vi "校准任务流程.vi"(9 "校准任务":T1[](array[typedef]), 10 "精度":dbl=4.0, 11 "模型":enum32{"线性", "多项式", "折线"}(ring)) -> ()   [LabVIEW 2016, in "斯坦道CODMn.lvlib"]
uses:
  <userlib>/_OpenG.lib/array/array.llb/Remove Duplicates from 1D Array (U16)__ogtk.vi
panel:
  out "元素":T1
  out "执行列表":T2(ring)
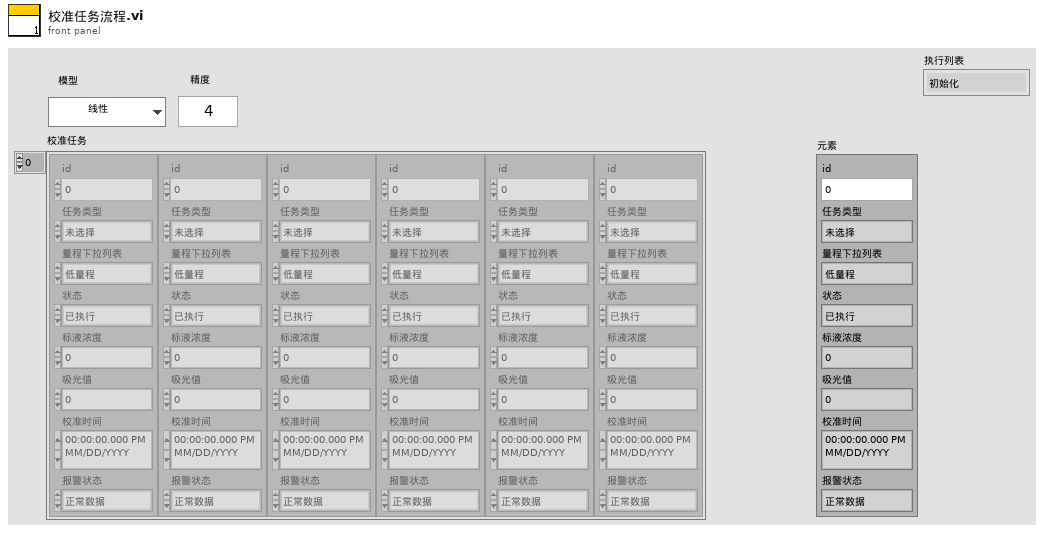
[diagram p1: front panel]
types:
  T1 = typedef "斯坦道CODMn.lvlib/校准任务.ctl" = cluster{"id":u16, "任务类型":enum16{"未选择", "空白校准", "标样校准", "标样核查", "零点核查", "跨度核查"}, "量程下拉列表":enum16{"低量程", "高量程"}, "状态":enum16{"已执行", "待执行", "执行中", "停止"}, "标液浓度":dbl, "吸光值":dbl, "校准时间":timestamp, "报警状态":enum16{"正常数据", "报警数据"}}
  T2 = enum16{"初始化", "解析数据", "判断任务类型", "执行测试任务", "等待测试任务完成", "获取测试数据", "任务结束判定", "计算公式", "结束"}
  T3 = cluster{"时间标识":timestamp, "设备":string, "日志信息":string, "流程参数":string}
  T4 = cluster{"测量模式":enum16{"水样测量", "标样核查", "零点核查", "跨度核查", "空白测试", "加标回收", "平行样", "校零", "校标"}}
  T5 = enum16{"水样测量", "标样核查", "零点核查", "跨度核查", "空白测试", "加标回收", "平行样", "校零", "校标"}
  T6 = cluster{"标液浓度1":dbl, "测量吸光度1":dbl, "样品1启用":bool, "标液浓度2":dbl, "测量吸光度2":dbl, "样品2启用":bool, "标液浓度3":dbl, "测量吸光度3":dbl, "样品3启用":bool, "标液浓度4":dbl, "测量吸光度4":dbl, "样品4启用":bool, "标液浓度5":dbl, "测量吸光度5":dbl, "样品5启用":bool, "模型":enum32{"线性", "多项式", "折线"}, "精度":dbl, "XY图":cluster{"X Values":dbl[], "Y Values":dbl[]}[], "拟合公式":string, "r^2":dbl, "标样一校准时间":timestamp, "标样二校准时间":timestamp, "标样三校准时间":timestamp, "标样四校准时间":timestamp, "标样五校准时间":timestamp, "二次方程":cluster{"c":dbl, "B":dbl, "x^2":dbl}, "标定时间":timestamp, "拟合公式 2":string, "r^2 2":dbl}
  T7 = enum16{"", "水样测量", "标样核查", "零点核查", "跨度核查", "空白测试", "平行样测试", "加标回收", "空白校准", "标样校准"}
  T8 = typedef "报警信息字段定义.ctl" = cluster{"时间":timestamp, "参数":string, "报警信息":string, "备注":string, "code":u64, "platform_alarm_code":string}
  T9 = cluster{"因子编码":u32, "单位":u16, "标样参考值":sgl, "水样数据时间":timestamp, "水样实测值":sgl, "水样数据标识":string, "标样数据时间":timestamp, "标样实测值":sgl, "标样数据标识":string, "空白数据时间":timestamp, "空白实测值":sgl, "空白数据标识":string, "零点核查数据时间":timestamp, "零点核查实测值":sgl, "零点核查数据标识":string, "跨度核查数据时间":timestamp, "跨度核查实测值":sgl, "跨度核查数据标识":string, "加标回收数据时间":timestamp, "加标回收实测值":sgl, "加标回收数据标识":string, "平行样数据时间":timestamp, "平行样实测值":sgl, "平行样数据标识":string}
  T10 = cluster{"时间":timestamp, "测量模式":string, "数据类型":string, "检测值":sgl, "单位":string, "数据标识":string, "因子编码":string, "标样参考值":sgl, "ORP-A":sgl, "ORP-B":sgl, "ORP-K":sgl, "COD滴定值":sgl, "高锰酸钾滴定数":sgl, "温度":sgl, "量程":sgl, "LastTime":timestamp, "序列号:":string, "跨度值":sgl, "高锰酸钾原始滴定数":sgl, "F0":sgl, "F1":sgl, "F2":sgl, "F3":sgl, "F4":sgl, "F5":sgl, "启动温度":sgl}
  T11 = enum16{"未选择", "空白校准", "标样校准", "标样核查", "零点核查", "跨度核查"}
  T12 = cluster{"标液浓度1":dbl, "测量吸光度1":dbl, "样品1启用":bool, "标液浓度2":dbl, "测量吸光度2":dbl, "样品2启用":bool, "标液浓度3":dbl, "测量吸光度3":dbl, "样品3启用":bool, "标液浓度4":dbl, "测量吸光度4":dbl, "样品4启用":bool, "标液浓度5":dbl, "测量吸光度5":dbl, "样品5启用":bool, "模型":enum32{"线性", "多项式", "折线"}, "精度":dbl, "XY图":cluster{"X Values":dbl[], "Y Values":dbl[]}[], "拟合公式":string, "r^2":dbl, "标样一校准时间":timestamp, "标样二校准时间":timestamp, "标样三校准时间":timestamp, "标样四校准时间":timestamp, "标样五校准时间":timestamp, "二次方程":cluster{"c":dbl, "x":dbl, "x^2":dbl}, "标定时间":timestamp, "拟合公式 2":string, "r^2 2":dbl}[][]
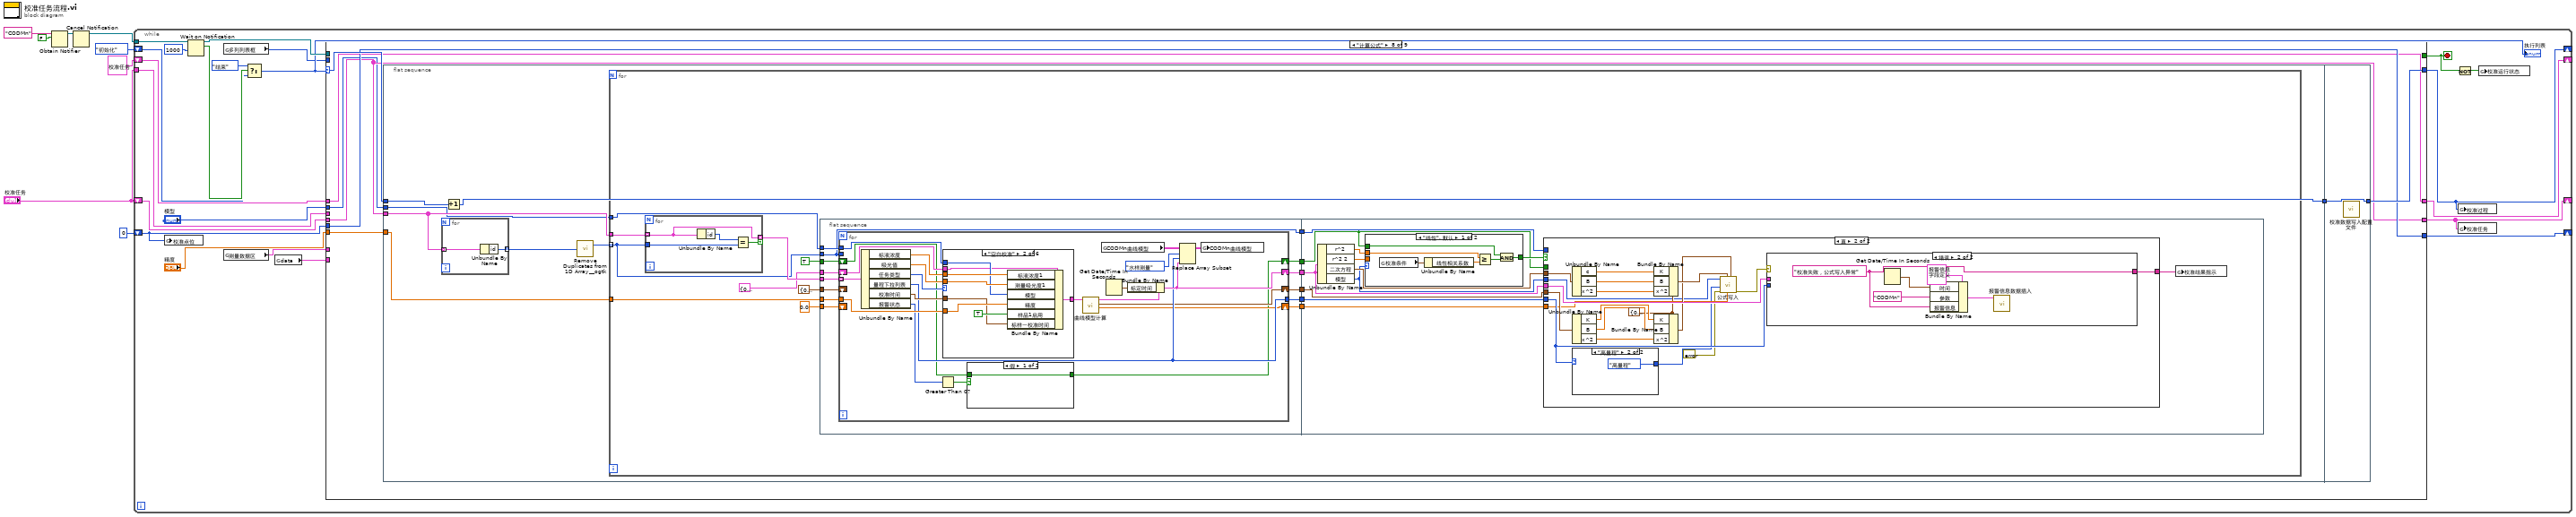
[diagram p0: block diagram]
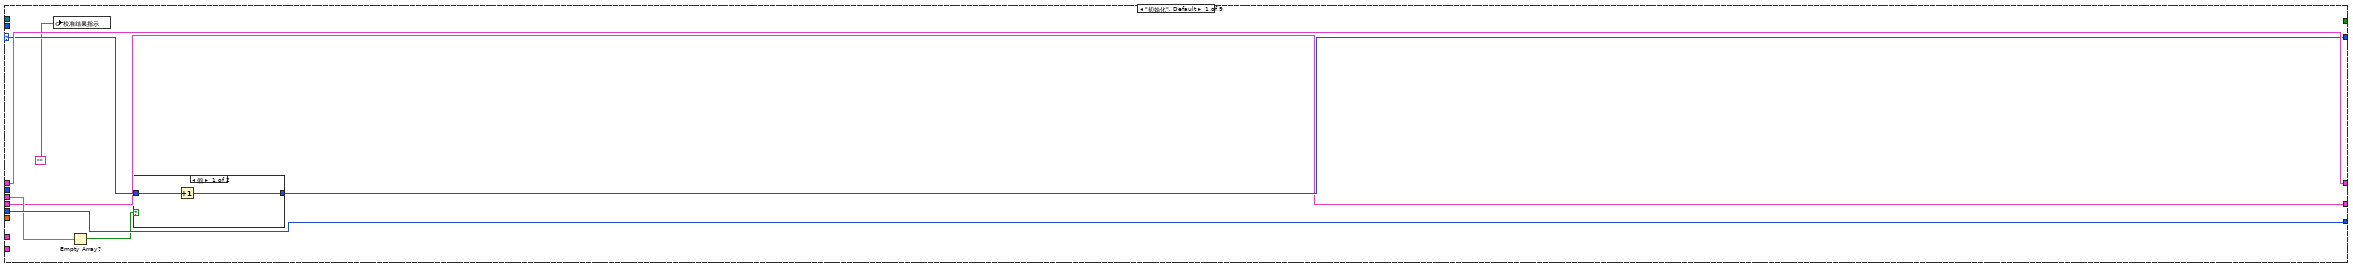
[diagram p2: hidden frame]
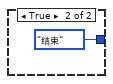
[diagram p3: hidden frame]
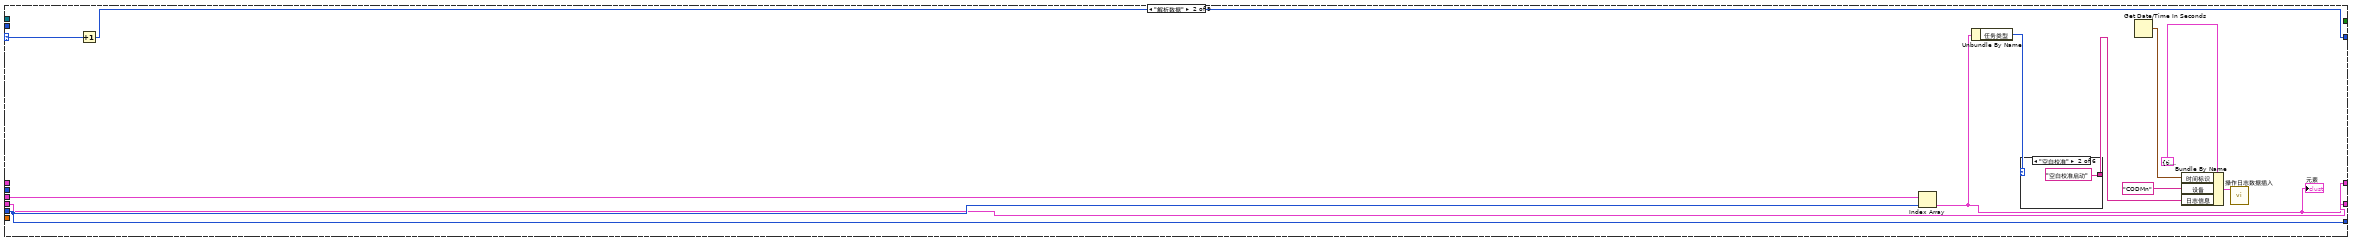
[diagram p4: hidden frame]
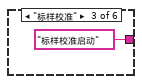
[diagram p6: hidden frame]
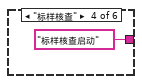
[diagram p7: hidden frame]
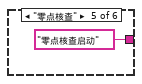
[diagram p8: hidden frame]
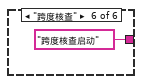
[diagram p9: hidden frame]
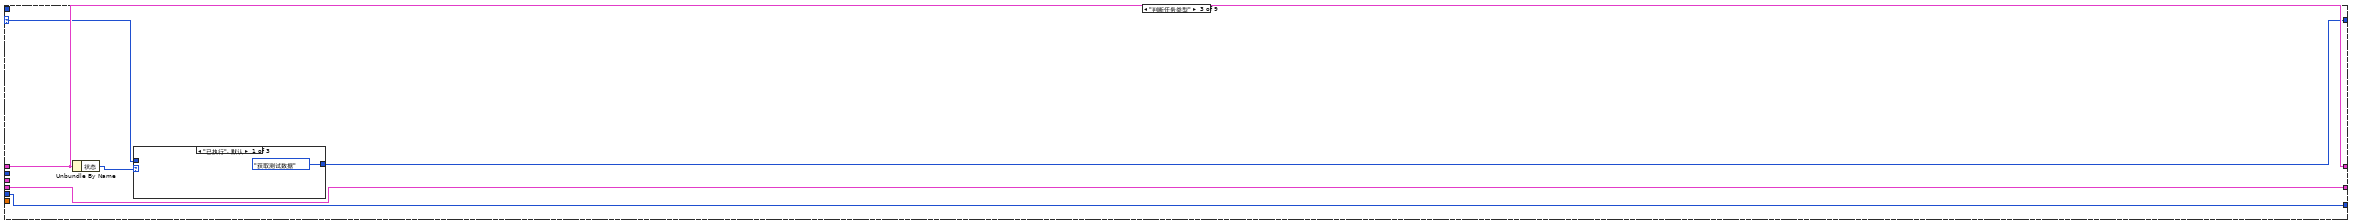
[diagram p10: hidden frame]
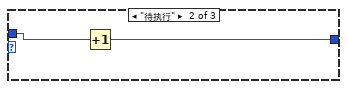
[diagram p11: hidden frame]
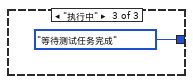
[diagram p12: hidden frame]
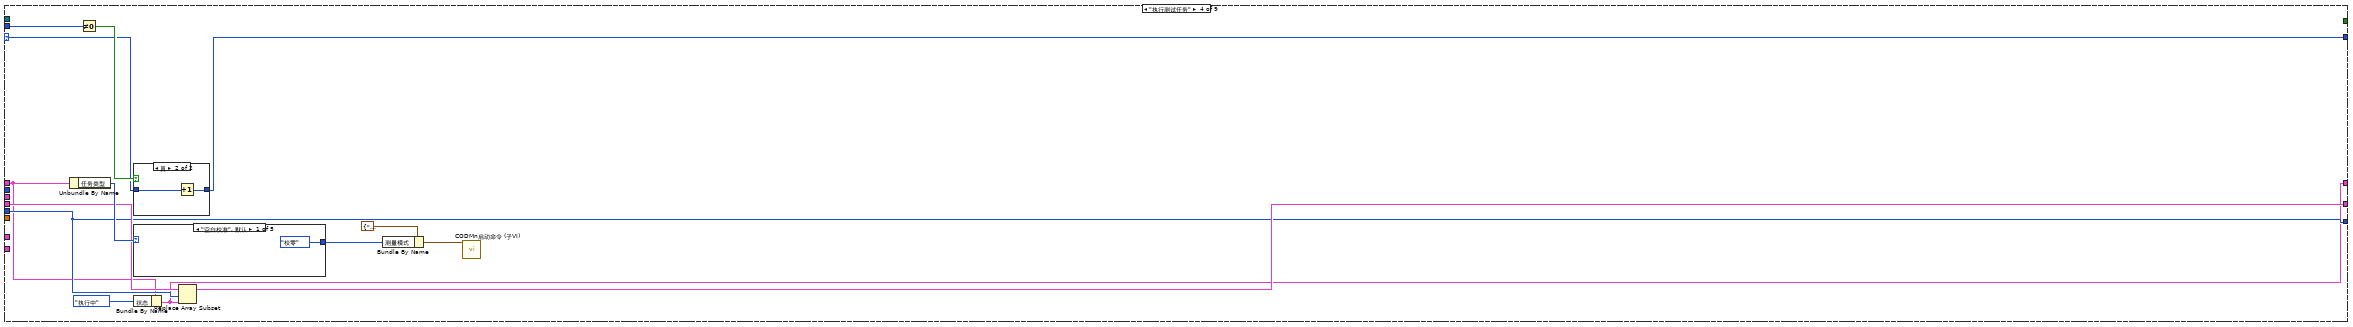
[diagram p13: hidden frame]
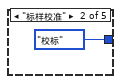
[diagram p15: hidden frame]
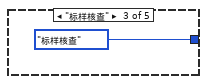
[diagram p16: hidden frame]
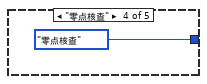
[diagram p17: hidden frame]
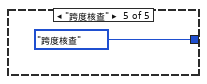
[diagram p18: hidden frame]
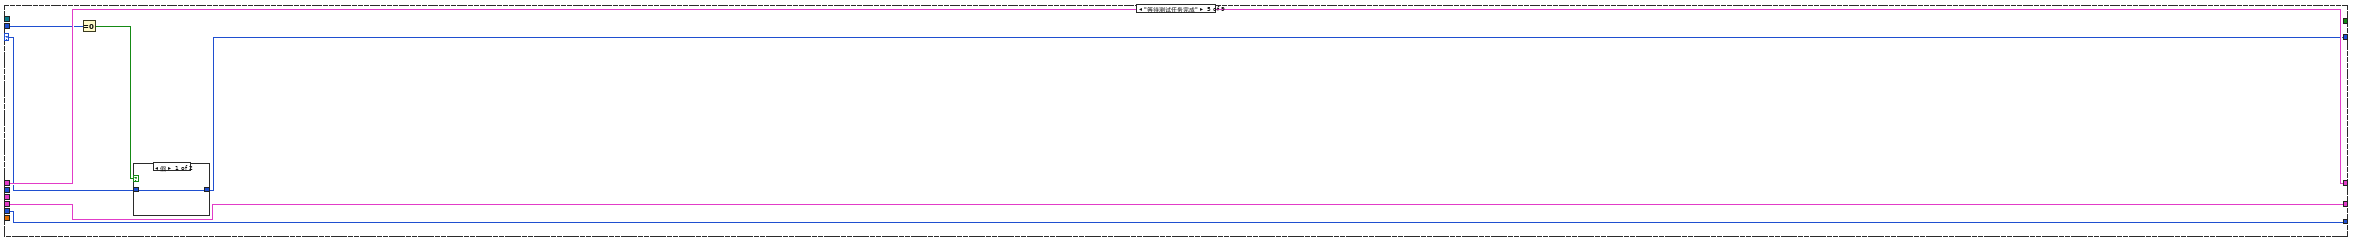
[diagram p19: hidden frame]
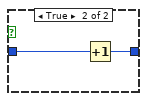
[diagram p20: hidden frame]
diagram:
  n1 = Obtain Notifier(name (unnamed)="CODMn" ("名称（未命名）"), notification data type=FALSE) -> (notifier out=w5:refnum<notifier>)  [unwired: 2 in, 2 out]
  n2 = Cancel Notification(0:w5) -> (8:w4:refnum<notifier>)  [unwired: 1 in, 2 out]
  n3 = while {
    shift-right: [w16] -> _
    shift-left: 0 -> [w12]
    shift-right: [w30] -> _
    shift-left: T1 {"id"=0, "任务类型"=enum."未选择", "量程下拉列表"=enum."低量程", "状态"=enum."待执行", "标液浓度"=0.0, "吸光值"=0.0, "校准时间"=timestamp(0 s since 1904-01-01), "报警状态"=enum."正常数据"} ("校准任务") -> [w29]
    shift-right: [w13] -> _
    shift-left: T2."初始化" ("执行列表") -> [w21]
    tunnel: w4 -> [w28]
    tunnel: "校准任务" -> [w27]
    shift-right: [w14] -> _
    shift-left: "校准任务" -> [w26]
    stop <- w17 stop-if-true
    n4 = global write "校准数据全局变量.vi" "校准点位"(w12) -> ()
    n5 = Wait on Notification(notifier=w28, timeout in ms (-1)=1000 ("超时毫秒(-1)")) -> (notifier out=w23:refnum<notifier>, notification=w22:bool)  [unwired: 2 in, 2 out]
    n6 = global read "运行时序全局变量.vi" "多列列表框"() -> (w11:i32)
    n7 = global read "CODMn断电保存全局变量.vi" "测量数据区"() -> (w10:T9)
    n8 = Select(t=T2."结束", s=w22, f=w21) -> (s? t:f=w20:T2)
    "执行列表" <- w20
    n9 = global read "COD内部交互全局.vi" "data"() -> (w9:T10)
    n10 = case shown="\"计算公式\"" w20 {
      selector: w20 -> [w36 w52 w61 w80 w95 w112 w159 w173 w352]
      tunnel: w12 -> [w37 w53 w63 w76 w96 w103 w160 w171 w350]
      tunnel: [w38 w46 w64 w73 w97 w107 w161 w170 w351] -> w30
      tunnel: w29 -> [w38 _ w64 w75 w97 w107 w161 w170 w351]
      tunnel: [w37 w53 w63 w76 w96 w103 w156 w171 w350] -> w16
      tunnel: [_ _ _ _ _ _ _ _ TRUE] -> w17
      tunnel: [w35 w51 w60 w79 w93 w111 w158 w172 w352] -> w13
      tunnel: w23 -> [_ _ _ _ _ _ _ _ w347]
      tunnel: w11 -> [_ _ _ w72 w91 w102 _ _ _]
      tunnel: w10 -> [_ _ _ _ _ w114 _ _ _]
      tunnel: w27 -> [w34 w50 _ _ _ _ w157 _ _]
      tunnel: [w33 w49 w59 w77 w92 w109 w153 w169 w348] -> w14
      tunnel: w26 -> [w33 w49 w59 w78 w92 w108 w153 w169 w348]
      tunnel: "模型" -> [_ _ _ _ _ _ _ w168 _]
      tunnel: "精度" -> [_ _ _ _ _ _ _ w167 _]
      tunnel: w9 -> [_ _ _ _ _ w101 _ _ _]
      frame "初始化", Default {
        n11 = global write "校准数据全局变量.vi" "校准结果指示"("") -> ()
        n12 = Empty Array?(array=w34) -> (empty?=w32:bool)
        n13 = case shown="假" w32 {
          tunnel: w36 -> [w40 _]
          tunnel: [w39 T2."结束"] -> w35
          frame False {
            n14 = Increment(x=w40) -> (x+1=w39:T2)
          }
          frame True {
          }
        }
      }
      frame "解析数据" {
        n15 = Increment(x=w52) -> (x+1=w51:T2)
        n16 = Index Array(array=w50, index=w53) -> (element=w46:T1)
        "元素" <- w46
        n17 = Unbundle By Name(w46) -> ("任务类型"=w45:T11)
        n18 = case shown="\"空白校准\"" w45 {
          tunnel: [_ "空白校准启动" "标样校准启动" "标样核查启动" "零点核查启动" "跨度核查启动"] -> w44
          frame "未选择", Default {
          }
          frame "空白校准" {
          }
          frame "标样校准" {
          }
          frame "标样核查" {
          }
          frame "零点核查" {
          }
          frame "跨度核查" {
          }
        }
        n19 = Get Date/Time In Seconds() -> (seconds since 1Jan1904=w48:timestamp)
        n20 = Bundle By Name(cluster=T3 {"时间标识"=timestamp(0 s since 1904-01-01), "设备"="", "日志信息"="", "流程参数"=""} ("data in"), "时间标识"=w48, "设备"="CODMn", "日志信息"=w44) -> (w43:T3)
        n21 = call "操作日志数据插入.vi"("data"=w43) -> ()  [unwired: 9 in, 1 out]
      }
      frame "判断任务类型" {
        n22 = Unbundle By Name(w64) -> ("状态"=w62:enum16{"已执行", "待执行", "执行中", "停止"})
        n23 = case shown="\"已执行\", 默认" w62 {
          tunnel: w61 -> [_ w67 _]
          tunnel: [T2."获取测试数据" w66 T2."等待测试任务完成"] -> w60
          frame "已执行", Default {
          }
          frame "待执行" {
            n24 = Increment(x=w67) -> (x+1=w66:T2)
          }
          frame "执行中" {
          }
        }
      }
      frame "执行测试任务" {
        n25 = Unbundle By Name(w75) -> ("任务类型"=w82:T11)
        n26 = Not Equal To 0?(x=w72) -> (x != 0?=w81:bool)
        n27 = case shown="真" w81 {
          tunnel: w80 -> [w83 w85]
          tunnel: [w83 w84] -> w79
          frame False {
          }
          frame True {
            n28 = Increment(x=w85) -> (x+1=w84:T2)
          }
        }
        n29 = case shown="\"空白校准\", 默认" w82 {
          tunnel: [T5."校零" ("测量模式") T5."校标" ("测量模式") T5."标样核查" ("测量模式") T5."零点核查" ("测量模式") T5."跨度核查" ("测量模式")] -> w69
          frame "空白校准", Default {
          }
          frame "标样校准" {
          }
          frame "标样核查" {
          }
          frame "零点核查" {
          }
          frame "跨度核查" {
          }
        }
        n30 = Bundle By Name(cluster=w75, "状态"=enum16{"已执行", "待执行", "执行中", "停止"}."执行中") -> (w73:T1)
        n31 = Replace Array Subset(array=w78, new element=w73, index=w76) -> (w77:T1[])
        n32 = Bundle By Name(cluster=T4 {"测量模式"=enum."水样测量"} ("启动测量模式"), "测量模式"=w69) -> (w70:T4)
        n33 = call "CODMn启动命令 (子VI).vi"("启动测量模式"=w70) -> ()  [unwired: 11 in]
      }
      frame "等待测试任务完成" {
        n34 = Equal To 0?(x=w91) -> (x = 0?=w94:bool)
        n35 = case shown="假" w94 {
          tunnel: w95 -> [w98 w100]
          tunnel: [w98 w99] -> w93
          frame False {
          }
          frame True {
            n36 = Increment(x=w100) -> (x+1=w99:T2)
          }
        }
      }
      frame "获取测试数据" {
        n37 = Unbundle By Name(w107) -> ("任务类型"=w113:T11, "状态"=w106:enum16{"已执行", "待执行", "执行中", "停止"})
        n38 = case shown="\"待执行\", 默认" w106 {
          tunnel: w114 -> [_ w127]
          tunnel: w113 -> [_ w126]
          tunnel: [w115 w124] -> w110
          tunnel: w107 -> [w115 w123]
          tunnel: w102 -> [_ w122]
          tunnel: w101 -> [_ w121]
          frame "已执行" {
          }
          frame "待执行", Default {
            n39 = case shown="\"标样校准\"" w126 {
              tunnel: w127 -> [w132 w137 w142 w147 w152]
              tunnel: [w131 w136 w141 w146 w151] -> w125
              tunnel: [w129 w134 w139 w144 w149] -> w116
              tunnel: w122 -> [_ _ _ _ _]
              tunnel: [w128 w133 w138 w143 w148] -> w120
              tunnel: w121 -> [w130 w135 w140 w145 w150]
              frame "空白校准", Default {
                n40 = Unbundle By Name(w130) -> ("高锰酸钾滴定数"=w129:sgl, "数据类型"=w128:string)
                n41 = Unbundle By Name(w132) -> ("空白数据时间"=w131:timestamp)
              }
              frame "标样校准" {
                n42 = Unbundle By Name(w135) -> ("高锰酸钾滴定数"=w134:sgl, "数据类型"=w133:string)
                n43 = Unbundle By Name(w137) -> ("标样数据时间"=w136:timestamp)
              }
              frame "标样核查" {
                n44 = Unbundle By Name(w140) -> ("高锰酸钾滴定数"=w139:sgl, "数据类型"=w138:string)
                n45 = Unbundle By Name(w142) -> ("标样数据时间"=w141:timestamp)
              }
              frame "零点核查" {
                n46 = Unbundle By Name(w147) -> ("零点核查数据时间"=w146:timestamp)
                n47 = Unbundle By Name(w145) -> ("高锰酸钾滴定数"=w144:sgl, "数据类型"=w143:string)
              }
              frame "跨度核查" {
                n48 = Unbundle By Name(w152) -> ("跨度核查数据时间"=w151:timestamp)
                n49 = Unbundle By Name(w150) -> ("高锰酸钾滴定数"=w149:sgl, "数据类型"=w148:string)
              }
            }
            n50 = Equal?(x=w120, y="D") -> (x = y?=w118:bool)
            n51 = Boolean To (0,1)(Boolean=w118) -> (0, 1=w117:i16)
            n52 = Bundle By Name(cluster=w123, "校准时间"=w125, "吸光值"=w116, "报警状态"=w117) -> (w124:T1)
          }
        }
        n53 = Increment(x=w112) -> (x+1=w111:T2)
        n54 = Bundle By Name(cluster=w110, "状态"=enum16{"已执行", "待执行", "执行中", "停止"}."已执行") -> (w104:T1)
        n55 = Replace Array Subset(array=w108, new element=w104, index=w103) -> (w109:T1[])
      }
      frame "任务结束判定" {
        n56 = Array Size(array=w157) -> (size(s)=w155:i32)
        n57 = Increment(x=w160) -> (x+1=w156:i32)
        n58 = Greater Or Equal?(x=w156, y=w155) -> (x >= y?=w154:bool)
        n59 = case shown="假" w154 {
          tunnel: w159 -> [_ w165]
          tunnel: [T2."解析数据" w164] -> w158
          frame False {
            n60 = Wait (ms)(milliseconds to wait=u32 3000 ("等待时间（毫秒）")) -> ()  [unwired: 1 out]
          }
          frame True {
            n61 = Increment(x=w165) -> (x+1=w164:T2)
          }
        }
      }
      frame "计算公式" {
        n62 = flat-sequence {
          tunnel: w173 -> [w180]
          tunnel: w169 -> [w176]
          tunnel: w168 -> [w175]
          tunnel: w167 -> [w174]
          tunnel: [w179] -> w166
          tunnel: [w346] -> w172
          tunnel: w166 -> [w346]
          frame #0 {
            n63 = for {
              tunnel: w176 -> [w345] mode=indexing
              tunnel: [w344] -> w178 mode=indexing
              n64 = Unbundle By Name(w345) -> ("id"=w344:u16)
            }
            n65 = Increment(x=w180) -> (x+1=w179:T2)
            n66 = call-poly <userlib>:"Remove Duplicates from 1D Array__ogtk.vi"("Input Array"=w178) -> ("Output Array"=w177:u16[])  [unwired: 1 out]
            n67 = for {
              tunnel: w177 -> [w193] mode=indexing
              tunnel: w176 -> [w195]
              tunnel: w175 -> [w192]
              tunnel: w174 -> [w191]
              n68 = for {
                tunnel: w195 -> [w341] mode=indexing
                tunnel: w193 -> [w343]
                tunnel: [w341] -> w194 mode=indexing if=w342
                n69 = Unbundle By Name(w341) -> ("id"=w340:u16)
                n70 = Equal?(x=w340, y=w343) -> (x = y?=w342:bool)
              }
              n71 = flat-sequence {
                tunnel: w194 -> [w208]
                tunnel: w193 -> [w203]
                tunnel: w192 -> [w207]
                tunnel: w191 -> [w206]
                tunnel: T6 {"标液浓度1"=0.0, "测量吸光度1"=0.0, "样品1启用"=FALSE, "标液浓度2"=0.0, "测量吸光度2"=0.0, "样品2启用"=FALSE, "标液浓度3"=0.0, "测量吸光度3"=0.0, "样品3启用"=FALSE, "标液浓度4"=0.0, "测量吸光度4"=0.0, "样品4启用"=FALSE, "标液浓度5"=0.0, "测量吸光度5"=0.0, "样品5启用"=FALSE, "模型"=enum."线性", "精度"=0.0, "XY图"=[], "拟合公式"="", "r^2"=0.0, "标样一校准时间"=timestamp(0 s since 1904-01-01), "标样二校准时间"=timestamp(0 s since 1904-01-01), "标样三校准时间"=timestamp(0 s since 1904-01-01), "标样四校准时间"=timestamp(0 s since 1904-01-01), "标样五校准时间"=timestamp(0 s since 1904-01-01), "二次方程"={"c"=0.0, "B"=0.0, "x^2"=0.0}, "标定时间"=timestamp(0 s since 1904-01-01), "拟合公式 2"="", "r^2 2"=0.0} ("输出簇") -> [w205]
                tunnel: [w204] -> w190
                tunnel: [w203] -> w189
                tunnel: [w202] -> w188
                tunnel: [w201] -> w187
                tunnel: cluster{"K":dbl, "B":dbl, "x^2":dbl} {"K"=0.0, "B"=0.0, "x^2"=0.0} ("二次方程 2") -> [w200]
                tunnel: [w199] -> w186
                tunnel: 0.0 ("公式切换阈值滴定数(0~9999)") -> [w198]
                tunnel: [w197] -> w184
                tunnel: TRUE -> [w196]
                tunnel: w190 -> [w282]
                tunnel: w189 -> [w284]
                tunnel: w188 -> [w283]
                tunnel: w187 -> [w281]
                tunnel: w186 -> [w280]
                tunnel: w184 -> [w276]
                frame #0 {
                  n72 = for {
                    tunnel: w208 -> [w230] mode=indexing
                    tunnel: w203 -> [_]
                    tunnel: w207 -> [w227]
                    tunnel: w206 -> [w226]
                    shift-right: [w220] -> w204
                    shift-left: w205 -> [w225]
                    tunnel: [w218] -> w202
                    shift-right: [w217] -> w201
                    shift-left: w200 -> [_]
                    shift-right: [w216] -> w199
                    shift-left: w198 -> [_]
                    shift-right: [w213] -> w197
                    shift-left: w196 -> [w211]
                    n73 = Unbundle By Name(w230) -> ("标液浓度"=w229:dbl, "吸光值"=w228:dbl, "任务类型"=w219:T11, "量程下拉列表"=w218:enum16{"低量程", "高量程"}, "校准时间"=w224:timestamp, "报警状态"=w214:enum16{"正常数据", "报警数据"})
                    n74 = Greater Than 0?(x=w214) -> (x > 0?=w212:bool)
                    n75 = case shown="\"空白校准\"" w219 {
                      tunnel: w229 -> [_ w241 w249 w257 w265 w273]
                      tunnel: w228 -> [_ w240 w242 w256 w264 w272]
                      tunnel: w227 -> [_ w239 w248 w255 w263 w271]
                      tunnel: w226 -> [_ w238 w247 w254 w262 w270]
                      tunnel: w225 -> [w233 w236 w245 w252 w260 w268]
                      tunnel: [w233 w234 w244 w251 w259 w267] -> w223
                      tunnel: w224 -> [_ w235 w243 w250 w258 w266]
                      frame "未选择", Default {
                        (unwired) T7."" ("测量模式")
                      }
                      frame "空白校准" {
                        n76 = Bundle By Name(cluster=w236, "标液浓度1"=w241, "测量吸光度1"=w240, "模型"=w239, "精度"=w238, "样品1启用"=TRUE, "标样一校准时间"=w235) -> (w234:T6)
                      }
                      frame "标样校准" {
                        (unwired) T7."标样校准" ("测量模式")
                        n77 = Bundle By Name(cluster=w245, "标液浓度2"=w249, "测量吸光度2"=w242, "模型"=w248, "精度"=w247, "样品2启用"=TRUE ("样品1启用"), "标样二校准时间"=w243) -> (w244:T6)
                      }
                      frame "标样核查" {
                        (unwired) T7."标样核查" ("测量模式")
                        n78 = Bundle By Name(cluster=w252, "标液浓度3"=w257, "测量吸光度3"=w256, "模型"=w255, "精度"=w254, "样品3启用"=TRUE ("样品1启用"), "标样三校准时间"=w250) -> (w251:T6)
                      }
                      frame "零点核查" {
                        (unwired) T7."零点核查" ("测量模式")
                        n79 = Bundle By Name(cluster=w260, "标液浓度4"=w265, "测量吸光度4"=w264, "模型"=w263, "精度"=w262, "样品4启用"=TRUE ("样品1启用"), "标样四校准时间"=w258) -> (w259:T6)
                      }
                      frame "跨度核查" {
                        (unwired) T7."跨度核查" ("测量模式")
                        n80 = Bundle By Name(cluster=w268, "标液浓度5"=w273, "测量吸光度5"=w272, "模型"=w271, "精度"=w270, "样品5启用"=TRUE ("样品1启用"), "标样五校准时间"=w266) -> (w267:T6)
                      }
                    }
                    n81 = case shown="假" w212 {
                      tunnel: [w231 FALSE] -> w213
                      tunnel: w211 -> [w231 _]
                      frame False {
                      }
                      frame True {
                      }
                    }
                    n82 = call "曲线模型计算.vi"("曲线模型"=w223) -> ("公式切换阈值滴定数(0~9999)"=w216:dbl, "二次方程 2"=w217:cluster{"K":dbl, "B":dbl, "x^2":dbl}, "输出簇"=w221:T6)  [unwired: 8 in]
                    n83 = global read "校准数据全局变量.vi" "CODMn曲线模型"() -> (w209:T12)
                    n84 = Get Date/Time In Seconds() -> (seconds since 1Jan1904=w222:timestamp)
                    n85 = Bundle By Name(cluster=w221, "标定时间"=w222) -> (w220:T6)
                    n86 = Replace Array Subset(array=w209, new element=w220, index (row)=T7."水样测量" ("测量模式"), index (col)=w218) -> (w210:T12)
                    n87 = global write "校准数据全局变量.vi" "CODMn曲线模型"(w210) -> ()
                  }
                }
                frame #1 {
                  n88 = Unbundle By Name(w282) -> ("r^2"=w279:dbl, "r^2 2"=w278:dbl, "二次方程"=w285:cluster{"c":dbl, "B":dbl, "x^2":dbl}, "模型"=w275:enum32{"线性", "多项式", "折线"})
                  n89 = case shown="\"线性\", 默认" w275 {
                    tunnel: w279 -> [w291 w295]
                    tunnel: w278 -> [_ w296]
                    tunnel: [w288 w297] -> w277
                    tunnel: w276 -> [w287 w293]
                    frame "线性", Default {
                      n90 = global read "CODMn断电保存全局变量.vi" "校准条件"() -> (w286:cluster{"线性相关系数":dbl})
                      n91 = Unbundle By Name(w286) -> ("线性相关系数"=w290:dbl)
                      n92 = Greater Or Equal?(x=w291, y=w290) -> (x >= y?=w289:bool)
                      n93 = And(x=w287, y=w289) -> (x .and. y?=w288:bool)
                    }
                    frame "折线" {
                      n94 = global read "CODMn断电保存全局变量.vi" "校准条件"() -> (w292:cluster{"线性相关系数":dbl})
                      n95 = Unbundle By Name(w292) -> ("线性相关系数"=w294:dbl)
                      n96 = Greater Or Equal?(x=w295, y=w294) -> (x >= y?=w299:bool)
                      n97 = Greater Or Equal?(x=w296, y=w294) -> (x >= y?=w298:bool)
                      n98 = Compound Arithmetic op=AND ("复合运算")(w299, w298, w293) -> (w297:bool)
                    }
                  }
                  n99 = case shown="真" w277 {
                    tunnel: w285 -> [_ w325]
                    tunnel: w284 -> [_ _]
                    tunnel: w283 -> [_ w316]
                    tunnel: w282 -> [_ w324]
                    tunnel: [w303 w323] -> w274
                    tunnel: w281 -> [_ w322]
                    tunnel: w280 -> [_ w315]
                    tunnel: w276 -> [w305 _]
                    tunnel: w275 -> [_ w312]
                    frame False {
                      n100 = case shown="假" w305 {
                        tunnel: ["有故障数据" ("格式字符串") "校准条件未满足" ("格式字符串")] -> w304
                        frame False {
                        }
                        frame True {
                        }
                      }
                      n101 = Format Into String(format string="校准失败，%s" ("格式字符串"), w304) -> (resulting string=w303:string)  [unwired: 2 in, 1 out]
                      n102 = Get Date/Time In Seconds() -> (seconds since 1Jan1904=w307:timestamp)
                      n103 = Bundle By Name(cluster=T8 {"时间"=timestamp(0 s since 1904-01-01), "参数"="", "报警信息"="", "备注"="", "code"=0, "platform_alarm_code"=""} ("data"), "时间"=w307, "参数"="CODMn" ("设备"), "报警信息"=w303) -> (w300:T8)
                      n104 = call "报警信息数据插入.vi"("data"=w300) -> ()  [unwired: 9 in, 1 out]
                    }
                    frame True {
                      w313 = cluster{"K":dbl, "B":dbl, "x^2":dbl} {"K"=0.0, "B"=0.0, "x^2"=0.0} ("二次方程 2")
                      n105 = Unbundle By Name(w325) -> ("c"=w326:dbl, "B"=w327:dbl, "x^2"=w328:dbl)
                      n106 = Unbundle By Name(w322) -> ("K"=w320:dbl, "B"=w319:dbl, "x^2"=w318:dbl)
                      n107 = case shown="\"高量程\"" w316 {
                        tunnel: [enum16{"低量程", "高量程"}."低量程" ("量程选择") enum16{"低量程", "高量程"}."高量程" ("量程选择")] -> w310
                        frame "低量程", Default {
                        }
                        frame "高量程" {
                        }
                      }
                      n108 = Bundle By Name(cluster=w313, "K"=w326, "B"=w327, "x^2"=w328) -> (w321:cluster{"K":dbl, "B":dbl, "x^2":dbl})
                      n109 = Bundle By Name(cluster=w313, "K"=w320, "B"=w319, "x^2"=w318) -> (w317:cluster{"K":dbl, "B":dbl, "x^2":dbl})
                      n110 = call "公式写入.vi"("公式 2"=w317, "公式切换阈值滴定数(0-9999)"=w315, "公式"=w321, "Error in"=errorcluster {"status"=FALSE, "code"=0, "source"=""} ("error out"), "量程选择"=w310, "模型"=w312) -> ("error out"=w314:errorcluster)  [unwired: 5 in]
                      n111 = case shown="错误" w314 {
                        tunnel: w316 -> [w334 _]
                        tunnel: w324 -> [w332 _]
                        tunnel: ["校准成功" w337] -> w323
                        frame No Error {
                          n112 = call "校准记录.vi"("曲线模型"=w332, "量程"=w334, "测量模式"="所有测量模式") -> ()  [unwired: 8 in, 1 out]
                        }
                        frame Error {
                          w337 = "校准失败，公式写入异常"
                          n113 = Get Date/Time In Seconds() -> (seconds since 1Jan1904=w338:timestamp)
                          n114 = Bundle By Name(cluster=T8 {"时间"=timestamp(0 s since 1904-01-01), "参数"="", "报警信息"="", "备注"="", "code"=0, "platform_alarm_code"=""} ("data"), "时间"=w338, "参数"="CODMn", "报警信息"=w337) -> (w335:T8)
                          n115 = call "报警信息数据插入.vi"("data"=w335) -> ()  [unwired: 9 in, 1 out]
                        }
                      }
                    }
                  }
                  n116 = global write "校准数据全局变量.vi" "校准结果指示"(w274) -> ()
                }
              }
            }
          }
          frame #1 {
            n117 = call "校准数据写入配置文件.vi"() -> ()  [unwired: 11 in, 1 out]
          }
        }
      }
      frame "结束" {
        n118 = Release Notifier(notifier=w347) -> ()  [unwired: 2 in, 3 out]
      }
    }
    n119 = Not(x=w17) -> (.not. x?=w15:bool)
    n120 = global write "校准数据全局变量.vi" "校准过程"(w13) -> ()
    n121 = global write "校准数据全局变量.vi" "校准任务"(w14) -> ()
    n122 = global write "校准数据全局变量.vi" "校准运行状态"(w15) -> ()
  }
